vi "Flattening of SGL arrays.vi"() -> ()   [LabVIEW 2017]
uses:
  JSONtext.lvlib
panel:
  in  "enable LabVIEW extensions?":bool=TRUE
  in  "Boolean":bool
  out "time":dbl format="%#_3p"
  out "JSON string":string
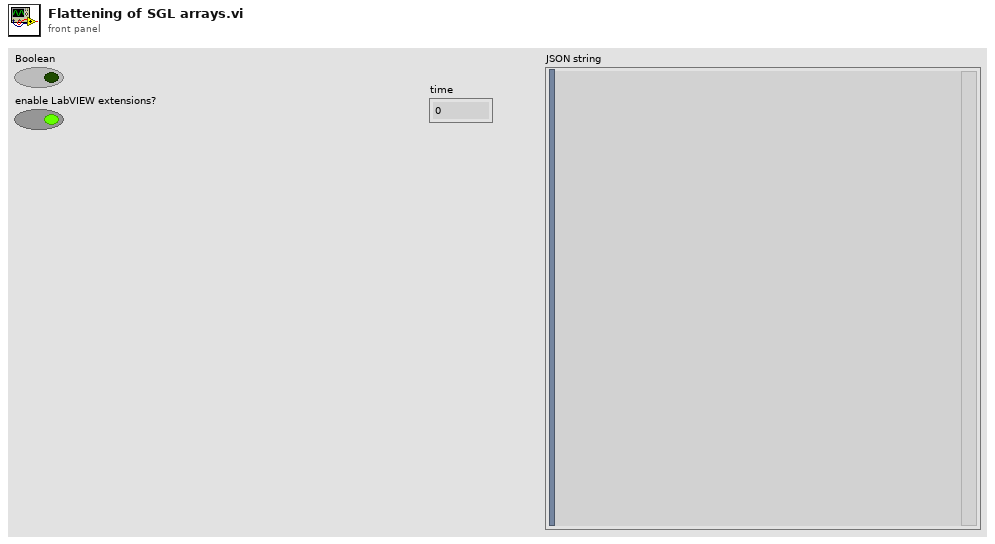
[diagram p1: front panel]
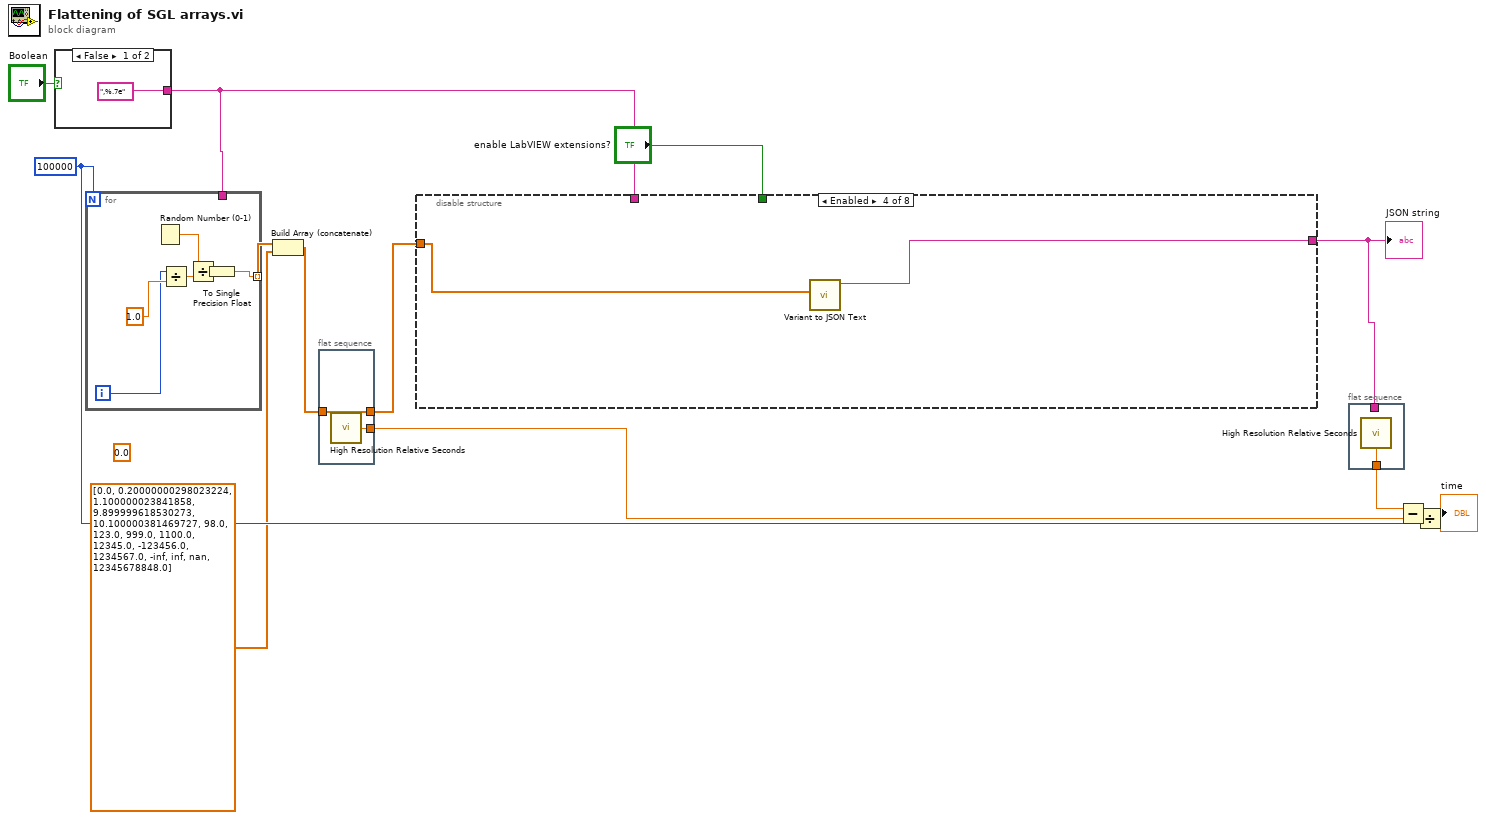
[diagram p0: block diagram]
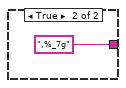
[diagram p2: hidden frame]
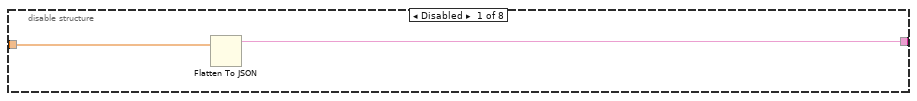
[diagram p3: hidden frame]
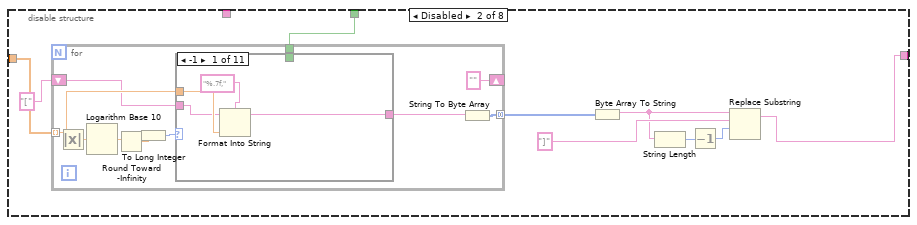
[diagram p4: hidden frame]
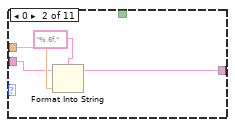
[diagram p5: hidden frame]
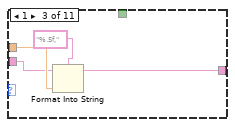
[diagram p6: hidden frame]
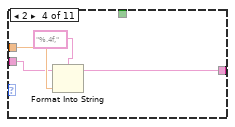
[diagram p7: hidden frame]
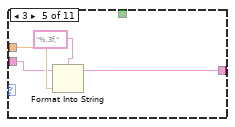
[diagram p8: hidden frame]
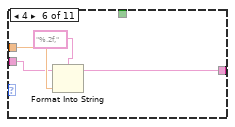
[diagram p9: hidden frame]
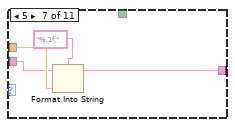
[diagram p10: hidden frame]
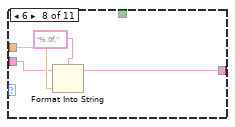
[diagram p11: hidden frame]
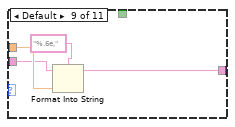
[diagram p12: hidden frame]
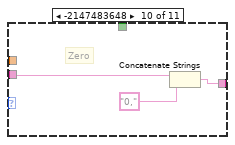
[diagram p13: hidden frame]
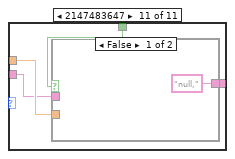
[diagram p14: hidden frame]
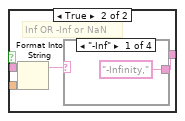
[diagram p15: hidden frame]
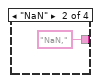
[diagram p16: hidden frame]
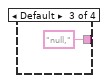
[diagram p17: hidden frame]
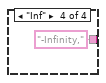
[diagram p18: hidden frame]
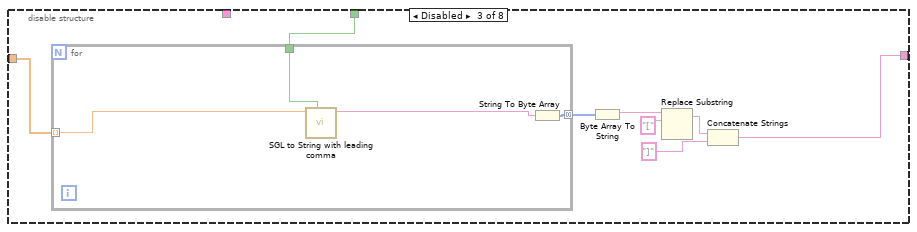
[diagram p19: hidden frame]
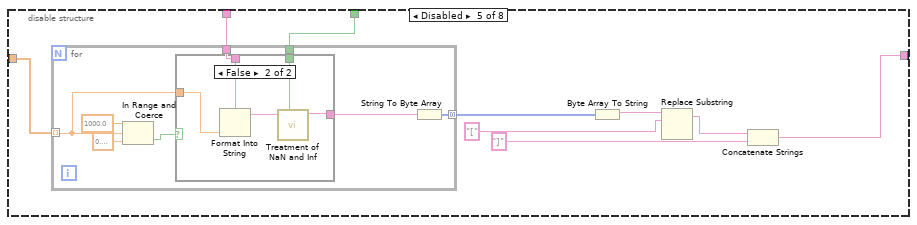
[diagram p20: hidden frame]
diagram:
  (unwired) sgl 0.0
  w6 = 100000
  n1 = case shown="False" "Boolean" {
    tunnel: [",%.7e" ("format string") ",%_7g" ("format string")] -> w3
    frame False {
    }
    frame True {
    }
  }
  n2 = for {
    N: w6 -> [_]
    tunnel: [w16] -> w10 mode=indexing
    tunnel: w3 -> [_]
    i -> [w17]
    n3 = Random Number (0-1)() -> (number: 0 to 1=w19:dbl)
    n4 = Divide(x=w17, y=1.0) -> (x/y=w20:dbl)
    n5 = Divide(x=w19, y=w20) -> (x/y=w18:dbl)
    n6 = To Single Precision Float(number=w18) -> (single precision float=w16:sgl)
  }
  n7 = Build Array (concatenate)(w10, sgl[] [0.0, 0.2, 1.1, 9.9, 10.1, 98.0, 123.0, 999.0, 1100.0, 12345.0, -123456.0, 1234567.0, -inf, inf, nan, 12345679000.0]) -> (w5:sgl[])
  n8 = flat-sequence {
    tunnel: [w23] -> w11
    tunnel: w5 -> [w22]
    tunnel: [w22] -> w9
    frame #0 {
      n9 = call <vilib>:"High Resolution Relative Seconds.vi"() -> ("relative seconds"=w23:dbl)
    }
  }
  n10 = disable-structure shown="Enabled" {
    disable-tunnel: [w25 w30 w98 w109 w113 w138 w153 w176] -> w13
    disable-tunnel: w9 -> [w24 w34 w104 w110 w119 w144 w163 w181]
    disable-tunnel: w3 -> [_ _ _ _ w112 w137 w151 _]
    disable-tunnel: "enable LabVIEW extensions?" -> [_ w32 w97 _ w111 w136 _ _]
    frame Disabled {
      n11 = Flatten To JSON(anything=w24) -> (JSON string=w25:string)  [unwired: 2 in, 1 out]
    }
    frame Disabled {
      n12 = for {
        tunnel: w34 -> [w42] mode=indexing
        tunnel: [w44] -> w33 mode=concatenating
        tunnel: w32 -> [w43]
        shift-right: [""] -> _
        shift-left: "[" -> [w37]
        n13 = Absolute Value(x=w42) -> (abs(x)=w38:sgl)
        n14 = Logarithm Base 10(1:w38) -> (0:w41:sgl)
        n15 = Round Toward -Infinity(1:w41) -> (0:w40:sgl)
        n16 = To Long Integer(number=w40) -> (32bit integer=w39:i32)
        n17 = case shown="-1" w39 {
          tunnel: [w48 w52 w56 w60 w64 w68 w72 w76 w79 w82 w87] -> w35
          tunnel: w42 -> [w47 w51 w55 w59 w63 w67 w71 w75 w80 _ w86]
          tunnel: w43 -> [_ _ _ _ _ _ _ _ _ _ w85]
          tunnel: w37 -> [w45 w49 w53 w57 w61 w65 w69 w73 w77 w81 w84]
          frame -1 {
            n18 = Format Into String(format string="%.7f,", initial string=w45, w47) -> (resulting string=w48:string)  [unwired: 1 in, 1 out]
          }
          frame 0 {
            n19 = Format Into String(format string="%.6f,", initial string=w49, w51) -> (resulting string=w52:string)  [unwired: 1 in, 1 out]
          }
          frame 1 {
            n20 = Format Into String(format string="%.5f,", initial string=w53, w55) -> (resulting string=w56:string)  [unwired: 1 in, 1 out]
          }
          frame 2 {
            n21 = Format Into String(format string="%.4f,", initial string=w57, w59) -> (resulting string=w60:string)  [unwired: 1 in, 1 out]
          }
          frame 3 {
            n22 = Format Into String(format string="%.3f,", initial string=w61, w63) -> (resulting string=w64:string)  [unwired: 1 in, 1 out]
          }
          frame 4 {
            n23 = Format Into String(format string="%.2f,", initial string=w65, w67) -> (resulting string=w68:string)  [unwired: 1 in, 1 out]
          }
          frame 5 {
            n24 = Format Into String(format string="%.1f,", initial string=w69, w71) -> (resulting string=w72:string)  [unwired: 1 in, 1 out]
          }
          frame 6 {
            n25 = Format Into String(format string="%.0f,", initial string=w73, w75) -> (resulting string=w76:string)  [unwired: 1 in, 1 out]
          }
          frame Default {
            n26 = Format Into String(format string="%.6e,", initial string=w77, w80) -> (resulting string=w79:string)  [unwired: 1 in, 1 out]
          }
          frame -2147483648 {
            # "Zero"
            n27 = Concatenate Strings(w81, "0,") -> (w82:string)
          }
          frame 2147483647 {
            n28 = case shown="False" w85 {
              tunnel: ["null," w92] -> w87
              tunnel: w86 -> [_ w90]
              tunnel: w84 -> [_ w89]
              frame False {
              }
              frame True {
                # "Inf OR -Inf or NaN"
                n29 = Format Into String(initial string=w89, w90) -> (resulting string=w91:string)  [unwired: 2 in, 1 out]
                n30 = case shown="\"-Inf\"" w91 {
                  tunnel: ["-Infinity," "NaN," "null," "-Infinity,"] -> w92
                  frame "-Inf" {
                  }
                  frame "NaN" {
                  }
                  frame Default {
                  }
                  frame "Inf" {
                  }
                }
              }
            }
          }
        }
        n31 = String To Byte Array(string=w35) -> (unsigned byte array=w44:u8[])
      }
      n32 = Byte Array To String(unsigned byte array=w33) -> (string=w28:string)
      n33 = String Length(string=w28) -> (length=w27:i32)
      n34 = Decrement(x=w27) -> (x-1=w26:i32)
      n35 = Replace Substring(3:w26, 4:"]" ("string"), 5:w28) -> (1:w30:string)  [unwired: 1 in, 1 out]
    }
    frame Disabled {
      n36 = for {
        tunnel: w104 -> [w105] mode=indexing
        tunnel: [w108] -> w103 mode=concatenating
        tunnel: w97 -> [w106]
        n37 = call "SGL to String with leading comma.vi"("enable LabVIEW extensions?"=w106, "SGL"=w105) -> ("SGL string (with leading comma)"=w107:string)  [unwired: 9 in]
        n38 = String To Byte Array(string=w107) -> (unsigned byte array=w108:u8[])
      }
      n39 = Byte Array To String(unsigned byte array=w103) -> (string=w102:string)
      n40 = Replace Substring(4:"[" ("substring (\"\")"), 5:w102) -> (1:w100:string)  [unwired: 2 in, 1 out]
      n41 = Concatenate Strings(w100, "]" ("string")) -> (w98:string)
    }
    frame Enabled {
      n42 = call "Variant to JSON Text.vi"("Variant"=w110) -> ("<JSON>"=w109:string)  [unwired: 8 in, 2 out]
    }
    frame Disabled {
      n43 = for {
        tunnel: w119 -> [w121] mode=indexing
        tunnel: [w127] -> w118 mode=concatenating
        tunnel: w112 -> [w126]
        tunnel: w111 -> [w120]
        n44 = In Range and Coerce(upper limit=sgl 1000.0, x=w121, lower limit=sgl 0.1) -> (In Range?=w122:bool)  [unwired: 1 out]
        n45 = case shown="False" w122 {
          tunnel: w126 -> [_ w135]
          tunnel: [w130 w132] -> w125
          tunnel: w121 -> [w129 w134]
          tunnel: w120 -> [_ w131]
          frame True {
            n46 = Format Into String(format string=",%.7f", w129) -> (resulting string=w130:string)  [unwired: 2 in, 1 out]
          }
          frame False {
            n47 = Format Into String(format string=w135, w134) -> (resulting string=w133:string)  [unwired: 2 in, 1 out]
            n48 = call "Treatment of NaN and Inf.vi"("enable LabVIEW extensions?"=w131, "Numeric Text"=w133) -> ("<JSON>"=w132:string)  [unwired: 9 in]
          }
        }
        n49 = String To Byte Array(string=w125) -> (unsigned byte array=w127:u8[])
      }
      n50 = Byte Array To String(unsigned byte array=w118) -> (string=w117:string)
      n51 = Replace Substring(4:"[" ("substring (\"\")"), 5:w117) -> (1:w115:string)  [unwired: 2 in, 1 out]
      n52 = Concatenate Strings(w115, "]" ("string")) -> (w113:string)
    }
    frame Disabled {
      n53 = for {
        tunnel: w144 -> [w150] mode=indexing
        tunnel: [w149] -> w143 mode=concatenating
        tunnel: w137 -> [w148]
        tunnel: w136 -> [w145]
        n54 = Format Into String(format string=w148, w150) -> (resulting string=w147:string)  [unwired: 2 in, 1 out]
        n55 = call "Treatment of NaN and Inf.vi"("enable LabVIEW extensions?"=w145, "Numeric Text"=w147) -> ("<JSON>"=w146:string)  [unwired: 9 in]
        n56 = String To Byte Array(string=w146) -> (unsigned byte array=w149:u8[])
      }
      n57 = Byte Array To String(unsigned byte array=w143) -> (string=w142:string)
      n58 = Replace Substring(4:"[" ("substring (\"\")"), 5:w142) -> (1:w140:string)  [unwired: 2 in, 1 out]
      n59 = Concatenate Strings(w140, "]" ("string")) -> (w138:string)
    }
    frame Disabled {
      n60 = for {
        tunnel: w163 -> [w167] mode=indexing
        tunnel: w151 -> [w166]
        tunnel: [w164] -> w162 mode=indexing
        n61 = Format Into String(format string=w166, w167) -> (resulting string=w165:string)  [unwired: 2 in, 1 out]
        n62 = case shown="\"-Inf\"" w165 {
          selector: w165 -> [_ _ w170]
          tunnel: ["Infinity" "-Infinity" w170] -> w164
          frame "Inf" {
          }
          frame "-Inf" {
          }
          frame Default {
          }
        }
      }
      n63 = Array To Spreadsheet String(delimiter (Tab)=",", array=w162, 3:"" ("format string")) -> (spreadsheet string=w154:string)
      n64 = String Length(string=w154) -> (length=w157:i32)
      n65 = Subtract(x=w157, y=2) -> (x-y=w155:i32)
      n66 = String Subset(string=w154, length (rest)=w155) -> (substring=w158:string)  [unwired: 1 in]
      n67 = Concatenate Strings("[" ("substring (\"\")"), w158, "]" ("substring (\"\")")) -> (w153:string)
    }
    frame Disabled {
      n68 = Array To Spreadsheet String(delimiter (Tab)=",", array=w181, 3:"%#_7g" ("format string")) -> (spreadsheet string=w174:string)
      n69 = String Length(string=w174) -> (length=w173:i32)
      n70 = Subtract(x=w173, y=2) -> (x-y=w171:i32)
      n71 = String Subset(string=w174, length (rest)=w171) -> (substring=w175:string)  [unwired: 1 in]
      n72 = Concatenate Strings("[" ("substring (\"\")"), w175, "]" ("substring (\"\")")) -> (w176:string)
    }
  }
  "JSON string" <- w13
  n73 = flat-sequence {
    tunnel: w13 -> [_]
    tunnel: [w182] -> w12
    frame #0 {
      n74 = call <vilib>:"High Resolution Relative Seconds.vi"() -> ("relative seconds"=w182:dbl)
    }
  }
  n75 = Subtract(x=w12, y=w11) -> (x-y=w8:dbl)
  n76 = Divide(x=w8, y=w6) -> (x/y=→"time":dbl)
